vi "picoquant_initialize_log.vi"(8 "error in (no error)":errorcluster, 11 "hydraharp in":refnum<class "hydraharp.lvclass">) -> (0 "error out":errorcluster, 3 "hydraharp out":refnum<class "hydraharp.lvclass">)   [LabVIEW 2015, in "hydraharp.lvclass"]
uses:
  hydraharp.lvclass
  hydraharp.lvclass/hydraharp.ctl
  hdf5_photon_record_logger/hdf5_photon_record_log.lvclass
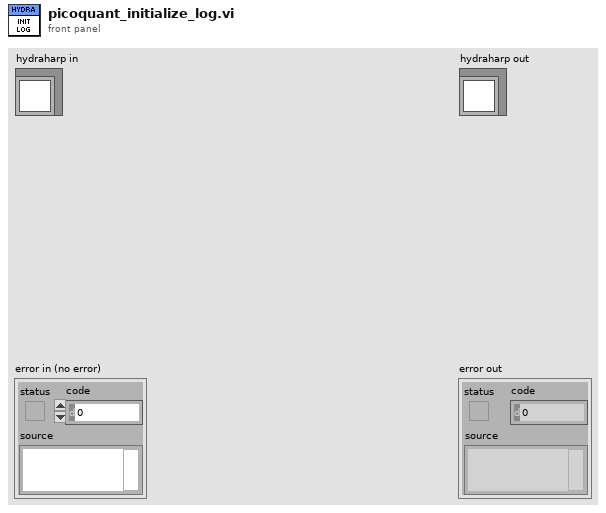
[diagram p1: front panel]
types:
  T1 = typedef "hpanel_acq_modes.ctl" = u16
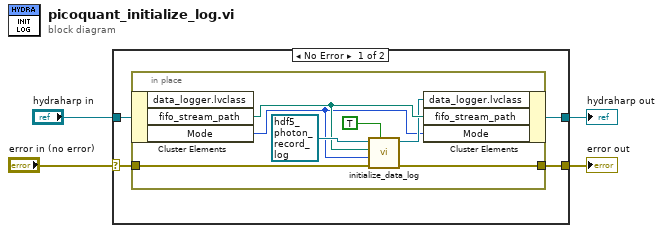
[diagram p0: block diagram]
diagram:
  n1 = case shown="No Error" "error in (no error)" {
    selector: "error in (no error)" -> [w7 w16]
    tunnel: "hydraharp in" -> [w8 w17]
    tunnel: [w6 w16] -> w2
    tunnel: [w5 w17] -> w1
    frame No Error {
      n2 = in-place {
        in-place-border: w7 -> [w12]
        in-place-border: [w11] -> w6
        n3 = in-place-cluster #1(w8) -> ("fifo_stream_path"=w13:path, "Mode"=w9:T1)  [unwired: 1 out]
        n4 = call-dynamic "initialize_data_log.vi"("Overwrite?"=TRUE, "error in (no error)"=w12, "Initialization Data"=w9, "Path"=w13, "hdf5_photon_record_log in"=refnum<class "hdf5_photon_record_log.lvclass"> refnum ("hdf5_photon_record_log.lvclass")) -> ("error out"=w11:errorcluster, "hdf5_photon_record_log out"=w10:refnum<class "hdf5_photon_record_log.lvclass">)  [unwired: 5 in]
        n5 = in-place-cluster #1("data_logger.lvclass"=w10, "fifo_stream_path"=w13, "Mode"=w9) -> (w5:refnum<class "hydraharp.lvclass">)
      }
    }
    frame Error {
    }
  }
  "error out" <- w2
  "hydraharp out" <- w1
